vi "CreateAndOpenTDMS.vi"(11 "Folder to save file to":path=path "C:/Users/LAV-UFSC-2023/Documents/LAV-TCC/Dados-Experimentos/Dados-Bancada-LABVIEW") -> (0 "error out":errorcluster, 1 "New file path":path, 3 "tdms file out":refnum<k34>)   [LabVIEW 2022 SP3]
uses:
  <vilib>/Utility/error.llb/DialogType.ctl
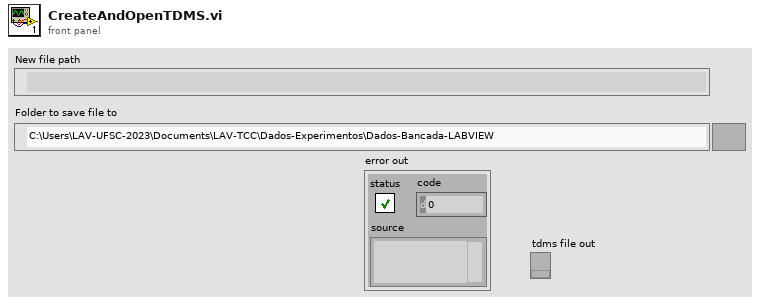
[diagram p1: front panel]
types:
  T1 = enum16{"open", "open or create", "create or replace", "create", "open (read-only)"}
  T2 = typedef "DialogType.ctl" = u16
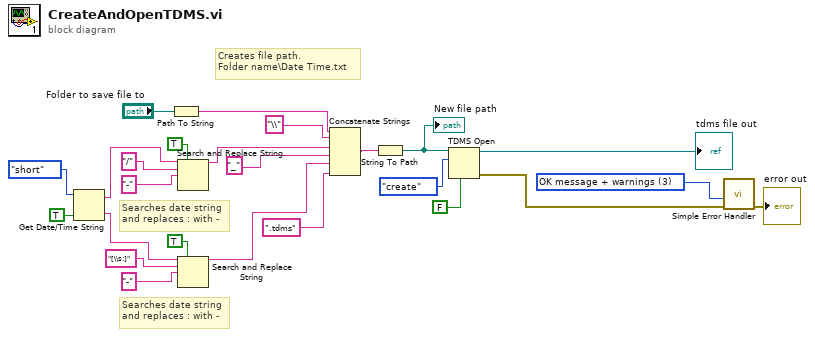
[diagram p0: block diagram]
diagram:
  w8 = T2 3 items=["no dialog", "OK message", "continue or stop message", "OK message + warnings", "continue/stop + warnings"] ("type of dialog (OK msg:1)")
  # "Searches date string\nand replaces : with -"
  # "Searches date string\nand replaces : with -"
  # "Creates file path.\nFolder name\\Date Time.txt"
  n1 = Get Date/Time String(date format (0)=enum16{"short", "long", "abbreviated"}."short", want seconds? (F)=TRUE) -> (date string=w10:string, time string=w23:string)  [unwired: 1 in]
  n2 = Path To String(path="Folder to save file to") -> (string=w18:string)
  n3 = Search and Replace String(replace all?=TRUE ("replace all? (F)"), input string=w10, search string="/" ("replace string (\"\")"), replace string="-" ("replace string (\"\")")) -> (result string=w9:string)  [unwired: 4 in, 3 out]
  n4 = Search and Replace String(replace all?=TRUE ("replace all? (F)"), input string=w23, search string="[\\s:]" ("replace string (\"\")"), replace string="-" ("replace string (\"\")")) -> (result string=w16:string)  [unwired: 4 in, 3 out]
  n5 = Concatenate Strings(w18, "\\" ("string"), w9, "_" ("string"), w16, ".tdms" ("string")) -> (w14:string)
  n6 = String To Path(string=w14) -> (path=w6:path)
  "New file path" <- w6
  n7 = TDMS Open(6:FALSE ("enable asynchronous? (T)"), 10:T1."create" ("operation (0:open)"), 11:w6) -> (0:w3:errorcluster, 3:→"tdms file out":refnum<k34>)  [unwired: 4 in]
  n8 = call <vilib>:"Simple Error Handler.vi"("type of dialog (OK msg:1)"=w8, "error in (no error)"=w3) -> ("error out"=→"error out":errorcluster)  [unwired: 3 in, 4 out]
